vi "TSM Sync Close Sessions.vi"(0 "TSM context":T1) -> (15 "error out":errorcluster)   [LabVIEW 2020]
doc: "Use this VI to reset and close all sessions for all NI-Sync instruments in the Semiconductor Module Context."
uses:
  <vilib>/NI_TestStand_SemiconductorModule/NI_TestStand_Semiconductor_Module.lvlibp/PinMap/General/SemiconductorModuleContext.ctl
  <vilib>/NI_TestStand_SemiconductorModule/NI_TestStand_Semiconductor_Module.lvlibp
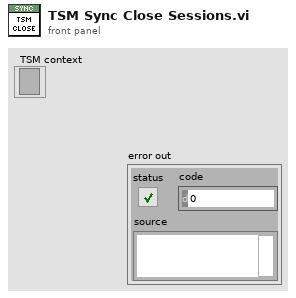
[diagram p1: front panel]
types:
  T1 = typedef "NI_TestStand_Semiconductor_Module.lvlibp/SemiconductorModuleContext.ctl" = refnum<k7>
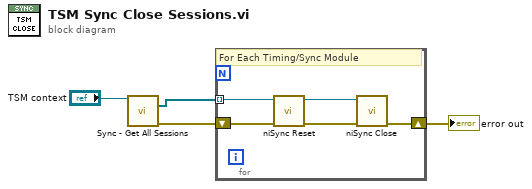
[diagram p0: block diagram]
diagram:
  n1 = call "Sync - Get All Sessions.vi"("TSM context"="TSM context") -> ("Sync Sessions Out"=w2:refnum<k15>[], "error out"=w4:errorcluster)  [unwired: 12 in, 1 out]
  n2 = for {
    tunnel: w2 -> [w8] mode=indexing
    shift-right: [w9] -> w1
    shift-left: w4 -> [w6]
    # "For Each Timing/Sync Module"
    n3 = call <instrlib>:"niSync Reset.vi"("error in (no error)"=w6, "instrument handle"=w8) -> ("error out"=w5:errorcluster, "instrument handle out"=w7:refnum<k15>)  [unwired: 8 in]
    n4 = call <instrlib>:"niSync Close.vi"("error in (no error)"=w5, "instrument handle"=w7) -> ("error out"=w9:errorcluster)  [unwired: 9 in]
  }
  "error out" <- w1
